vi "SS2 Live_Write HDF5 Header.vi"(8 "error in (no error)":errorcluster, 10 "Current Data Set":i32, 11 "ref in":T1 format="%.0x") -> (0 "Error Out":errorcluster, 1 "Notebook Message":string, 2 "# Image Sets":u32, 3 "ref out":T1 format="%.0x", 5 "# Data Sets":i32)   [LabVIEW 2019]
uses:
  <vilib>/addons/h5labview2/base/hid_t.ctl
  SS2 Live_Settings List.ctl
  SS2 Live_File Information.ctl
  SS2 Live_Image ROI Information.ctl
  Phasor/Image Binning Options.ctl
  SS2 DAQ Parameters 2.ctl
  SS2 Gate Definition.ctl
  Phasor/Fluorescence Lifetime Parameters.ctl
  <vilib>/addons/h5labview2/base/lib_path.vi
  <vilib>/addons/h5labview2/base/H5Equery.vi
  <vilib>/addons/h5labview2/dataset/H5Dwrite.llb/H5Dwrite.xnode
  <vilib>/addons/h5labview2/group/H5G.lvlib
  Variant/Variant to Data/Variant to Data.lvlib
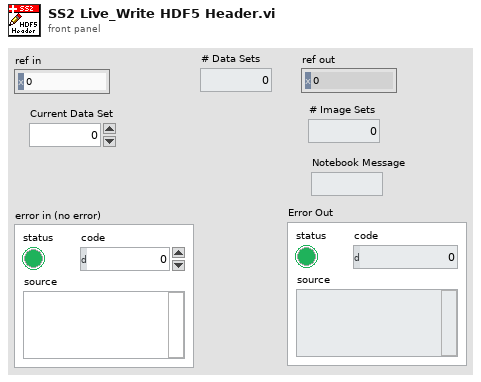
[diagram p1: front panel]
types:
  T1 = typedef "hid_t.ctl" = i32
  T2 = typedef "SS2 Live_Settings List.ctl" = enum16{"FPGA:Bitfile Path", "FPGA:Bitfile Version", "Acquisition Parameters:SS2 DAQ Parameters", "Acquisition Parameters:Gate Configuration Array", "Acquisition Parameters:Buffer Size (# Gates)", "File Information:File Information", "File Information:# Datasets in Series", "Image Parameters:Image ROI Information", "Image Parameters:Image Binning Options", "UI Parameters:Histogram Bins Number"}
  T3 = typedef "SS2 Live_File Information.ctl" = cluster{"File Folder":path, "File Name":string, "File Index":u32, "Author":string, "Sample":string, "Compression":bool}
  T4 = typedef "Image Binning Options.ctl" = cluster{"Use Image Binning":bool, "X Bin":i32, "Y Bin":i32}
  T5 = typedef "SS2 Live_Image ROI Information.ctl" = cluster{"Save ROI Only":bool, "Left":u16, "Top":u16, "Right":u16, "Bottom":u16, "Use Current ROI":bool}
  T6 = typedef "Fluorescence Lifetime Parameters.ctl" = cluster{"# Pixel X":i32, "# Pixel Y":i32, "# Gates":i32, "# Datasets":i32, "Exposure/Gate":dbl[unit], "Macrotime Gate Separation":dbl[unit], "Nanotime Gate Separation":dbl[unit], "Gate Duration":dbl[unit], "Laser Period":dbl[unit]}
  T7 = typedef "SS2 DAQ Parameters 2.ctl" = cluster{"10 bits":bool, "# Exposure Sequences":u32, "# 1-bit Frame per Gate":u32, "Gate Shift":u32, "# Gates per Set":u32, "# Sets":u32, "Laser Period":dbl[unit], "Gate Offset":u32, "Auto-adjust Gate Offset":bool, "Gate Definition":T8}
  T8 = typedef "SS2 Gate Definition.ctl" = cluster{"gs_psincdec_0":u32, "gs_psincdec_1":u32, "gs_psincdec_2":u32, "gs_psincdec_3":u32, "gs_no_shift_adj_1":u32, "gs_no_shift_adj_2":u32, "gs_no_shift_adj_3":u32}
  T9 = typedef "SS2 Live_Gate Characteristics.ctl" = cluster{"Predicted Gate Width":dbl[unit], "Gate Image Duration":dbl[unit], "Gate Image Exposure":dbl[unit], "Gate Shift":dbl[unit], "Gate Images Span":dbl[unit]}
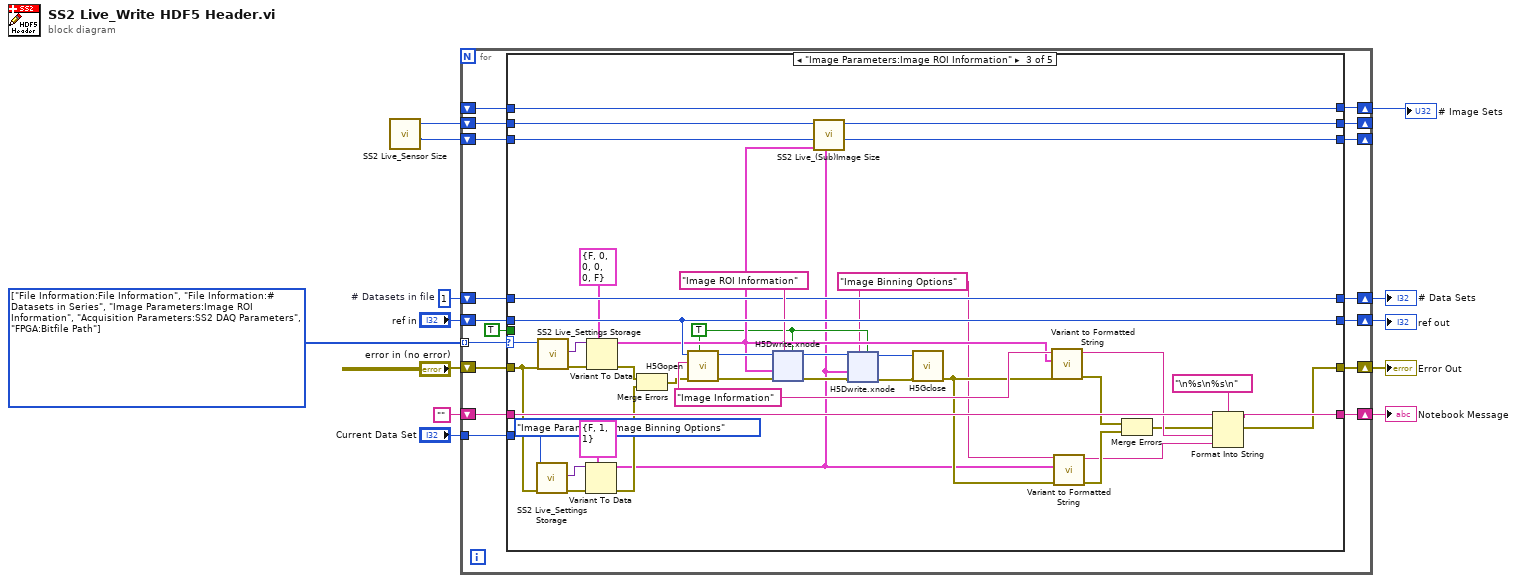
[diagram p0: block diagram]
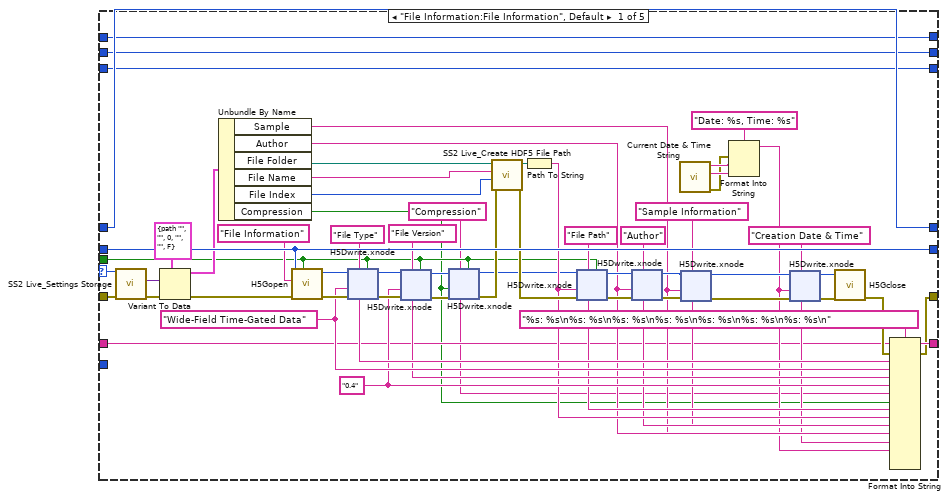
[diagram p2: hidden frame]
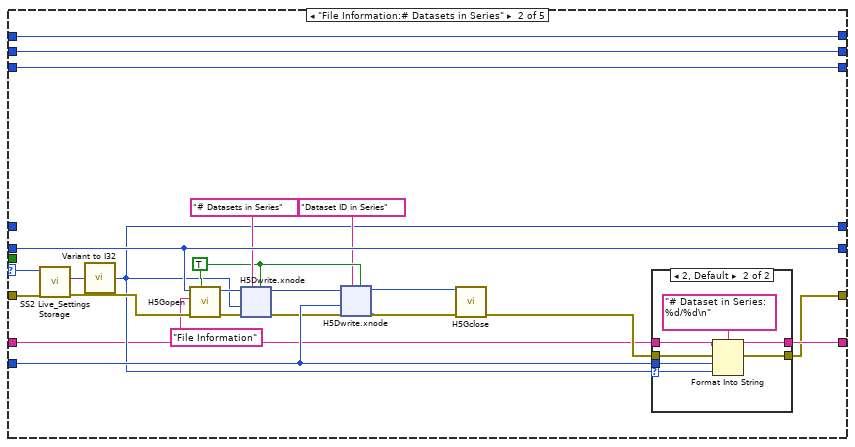
[diagram p3: hidden frame]
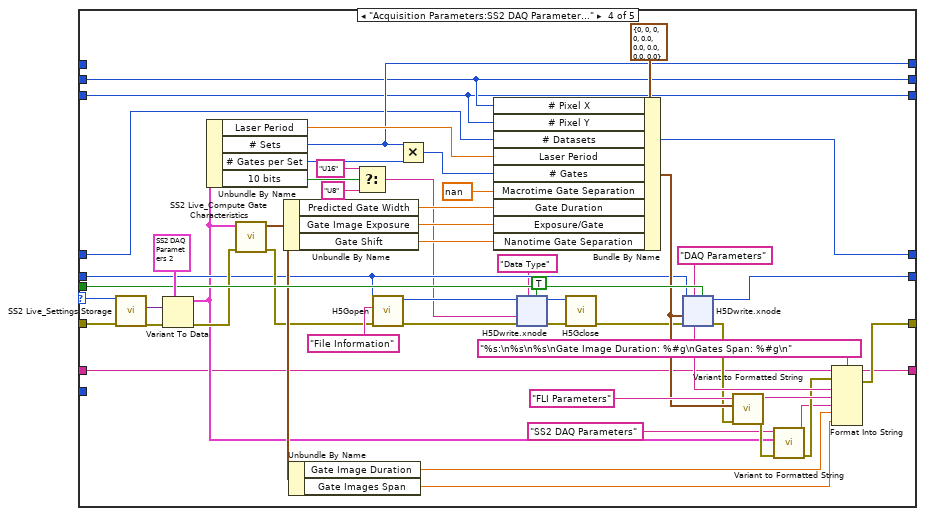
[diagram p5: hidden frame]
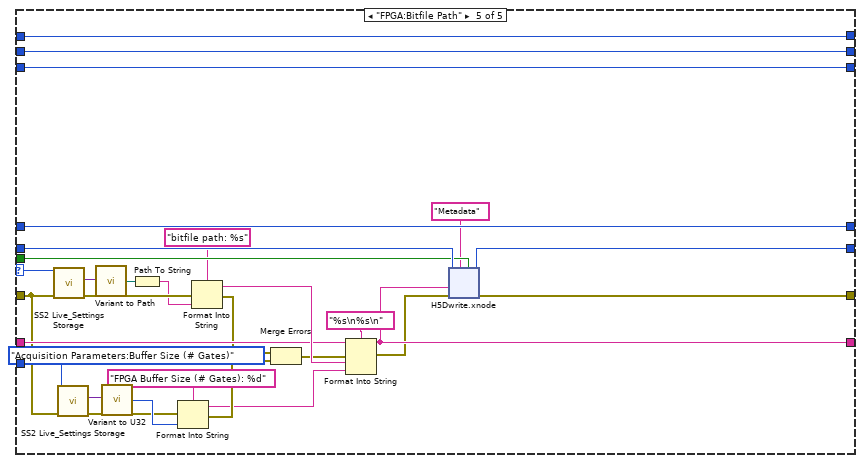
[diagram p6: hidden frame]
diagram:
  w8 = 1  # # Datasets in file
  w13 = T2[] [enum."File Information:File Information", enum."File Information:# Datasets in Series", enum."Image Parameters:Image ROI Information", enum."Acquisition Parameters:SS2 DAQ Parameters", enum."FPGA:Bitfile Path"] items=["FPGA:Bitfile Path", "FPGA:Bitfile Version", "Acquisition Parameters:SS2 DAQ Parameters", "Acquisition Parameters:Gate Configuration Array", "Acquisition Parameters:Buffer Size (# Gates)", "File Information:File Information", "File Information:# Datasets in Series", "Image Parameters:Image ROI Information", "Image Parameters:Image Binning Options", "UI Parameters:Histogram Bins Number"] ("Array")
  n1 = call "SS2 Live_Sensor Size.vi"() -> ("Y size"=w1:i32, "X size"=w2:i32)  [unwired: 10 in]
  n2 = for {
    tunnel: w13 -> [w30] mode=indexing
    shift-right: [w26] -> w10
    shift-left: "ref in" -> [w28]
    shift-right: [w27] -> w9
    shift-left: "error in (no error)" -> [w29]
    shift-right: [w23] -> w5
    shift-left: w8 -> [w22]
    tunnel: "Current Data Set" -> [w21]
    shift-right: [w20] -> w6
    shift-left: _ -> [w19]
    shift-right: [w24] -> w3
    shift-left: "" -> [w18]
    shift-right: [w16] -> _
    shift-left: w2 -> [w17]
    shift-right: [w14] -> _
    shift-left: w1 -> [w15]
    n3 = case shown="\"Image Parameters:Image ROI Information\"" w30 {
      selector: w30 -> [w84 w242 w331 w416 w488]
      tunnel: w29 -> [w85 w243 w302 w417 w466]
      tunnel: w28 -> [w79 w236 w329 w387 w485]
      tunnel: [w43 w239 w317 w404 w470] -> w27
      tunnel: [w79 w236 w329 w415 w484] -> w26
      tunnel: TRUE ("replace? (F)") -> [w33 _ _ w414 w483]
      tunnel: [w46 w240 w319 w374 w473] -> w24
      tunnel: [w42 w223 w324 w372 w477] -> w23
      tunnel: w22 -> [w42 _ w324 w372 w477]
      tunnel: w21 -> [_ w235 _ _ _]
      tunnel: [w41 w224 w325 w380 w476] -> w20
      tunnel: w19 -> [w41 w224 w325 _ w476]
      tunnel: w18 -> [w40 w222 w320 w373 w474]
      tunnel: [w39 w221 w312 w371 w469] -> w16
      tunnel: w17 -> [w39 w221 w313 w371 w469]
      tunnel: [w38 w220 w310 w370 w468] -> w14
      tunnel: w15 -> [w38 w220 w311 w370 w468]
      frame "File Information:File Information", Default {
        w32 = "Compression" ("dataset name")
        w48 = "Creation Date & Time" ("dataset name")
        w50 = "Sample Information" ("dataset name")
        w52 = "Author" ("dataset name")
        w54 = "File Path" ("dataset name")
        w57 = "Wide-Field Time-Gated Data" ("dataset name")
        w58 = "File Type" ("dataset name")
        w55 = "0.4" ("dataset name")
        w56 = "File Version" ("dataset name")
        n4 = call "SS2 Live_Settings Storage.vi"("Error In"=w85, "Settings List"=w84) -> ("Error Out"=w88:errorcluster, "Variant Data out"=w87:variant)  [unwired: 8 in]
        n5 = Variant To Data(error in=w88, type=T3 {"File Folder"=path "", "File Name"="", "File Index"=0, "Author"="", "Sample"="", "Compression"=FALSE} ("File Information"), Variant=w87) -> (data=w77:T3, error out=w78:errorcluster)
        n6 = Unbundle By Name(w77) -> ("Sample"=w49:string, "Author"=w51:string, "File Folder"=w76:path, "File Name"=w75:string, "File Index"=w74:u32, "Compression"=w31:bool)
        n7 = call <vilib>:"H5Gopen.vi"("create? (F)"=w33, "error in (no error)"=w78, "name"="File Information", "ref in"=w79) -> ("error out"=w82:errorcluster, "group out"=w83:T1)  [unwired: 6 in]
        n8 = xnode "H5Dwrite.xnode"("replace? (F)"=w33, "dataset name"=w58, "error in (no error)"=w82, "data"=w57, "ref in"=w83) -> ("error out"=w81:errorcluster, "ref out"=w80:i32)  [unwired: 2 in, 1 out]
        n9 = xnode "H5Dwrite.xnode"("replace? (F)"=w33, "dataset name"=w56, "error in (no error)"=w81, "data"=w55, "ref in"=w80) -> ("error out"=w37:errorcluster, "ref out"=w35:i32)  [unwired: 2 in, 1 out]
        n10 = xnode "H5Dwrite.xnode"("replace? (F)"=w33, "dataset name"=w32, "error in (no error)"=w37, "data"=w31, "ref in"=w35) -> ("error out"=w36:errorcluster, "ref out"=w34:i32)  [unwired: 2 in, 1 out]
        n11 = call "SS2 Live_Create HDF5 File Path.vi"("error in (no error)"=w36, "File Index"=w74, "File Name"=w75, "File Folder"=w76) -> ("error out"=w73:errorcluster, "File path"=w72:path)  [unwired: 6 in]
        n12 = Path To String(path=w72) -> (string=w53:string)
        n13 = xnode "H5Dwrite.xnode"("replace? (F)"=w33, "dataset name"=w54, "error in (no error)"=w73, "data"=w53, "ref in"=w34) -> ("error out"=w70:errorcluster, "ref out"=w71:i32)  [unwired: 2 in, 1 out]
        n14 = xnode "H5Dwrite.xnode"("dataset name"=w52, "error in (no error)"=w70, "data"=w51, "ref in"=w71) -> ("error out"=w69:errorcluster, "ref out"=w68:i32)  [unwired: 3 in, 1 out]
        n15 = call "Current Date & Time String.vi"() -> ("Error Out"=w62:errorcluster, "time string"=w63:string, "date string"=w64:string)  [unwired: 9 in]
        n16 = xnode "H5Dwrite.xnode"("dataset name"=w50, "error in (no error)"=w69, "data"=w49, "ref in"=w68) -> ("error out"=w67:errorcluster, "ref out"=w66:i32)  [unwired: 3 in, 1 out]
        n17 = Format Into String(format string="Date: %s, Time: %s", error in=w62, w64, w63) -> (resulting string=w47:string)  [unwired: 1 in, 1 out]
        n18 = xnode "H5Dwrite.xnode"("dataset name"=w48, "error in (no error)"=w67, "data"=w47, "ref in"=w66) -> ("error out"=w45:errorcluster, "ref out"=w65:i32)  [unwired: 3 in, 1 out]
        n19 = call <vilib>:"H5Gclose.vi"("error in (no error)"=w45, "group in"=w65) -> ("error out"=w44:errorcluster)  [unwired: 9 in]
        n20 = Format Into String(format string="%s: %s\n%s: %s\n%s: %s\n%s: %s\n%s: %s\n%s: %s\n%s: %s\n", initial string=w40, error in=w44, w58, w57, w56, w55, w32, w31, w54, w53, w52, w51, w50, w49, w48, w47) -> (resulting string=w46:string, error out=w43:errorcluster)
      }
      frame "File Information:# Datasets in Series" {
        w226 = TRUE ("replace? (F)")
        n21 = call "SS2 Live_Settings Storage.vi"("Error In"=w243, "Settings List"=w242) -> ("Error Out"=w238:errorcluster, "Variant Data out"=w241:variant)  [unwired: 8 in]
        n22 = call "Variant to I32.vi"("Variant"=w241) -> ("Value"=w223:i32)  [unwired: 8 in]
        n23 = call <vilib>:"H5Gopen.vi"("create? (F)"=w226, "error in (no error)"=w238, "name"="File Information", "ref in"=w236) -> ("error out"=w233:errorcluster, "group out"=w234:T1)  [unwired: 6 in]
        n24 = xnode "H5Dwrite.xnode"("replace? (F)"=w226, "dataset name"="# Datasets in Series" ("name"), "error in (no error)"=w233, "data"=w223, "ref in"=w234) -> ("error out"=w230:errorcluster, "ref out"=w228:i32)  [unwired: 2 in, 1 out]
        n25 = xnode "H5Dwrite.xnode"("replace? (F)"=w226, "dataset name"="Dataset ID in Series" ("name"), "error in (no error)"=w230, "data"=w235, "ref in"=w228) -> ("error out"=w229:errorcluster, "ref out"=w227:i32)  [unwired: 2 in, 1 out]
        n26 = call <vilib>:"H5Gclose.vi"("error in (no error)"=w229, "group in"=w227) -> ("error out"=w237:errorcluster)  [unwired: 9 in]
        n27 = case shown="2, Default" w223 {
          selector: w223 -> [_ w286]
          tunnel: [w282 w289] -> w240
          tunnel: w237 -> [w283 w288]
          tunnel: [w283 w287] -> w239
          tunnel: w235 -> [_ w285]
          tunnel: w222 -> [w282 w284]
          frame 0, 1 {
          }
          frame 2, Default {
            n28 = Format Into String(format string="# Dataset in Series: %d/%d\n", initial string=w284, error in=w288, w285, w286) -> (resulting string=w289:string, error out=w287:errorcluster)
          }
        }
      }
      frame "Image Parameters:Image ROI Information" {
        w294 = "Image Binning Options" ("name")
        w304 = TRUE ("replace? (F)")
        w316 = "Image Information" ("name")
        n29 = call "SS2 Live_Settings Storage.vi"("Error In"=w302, "Settings List"=SS2_Live_Settings_List."Image Parameters:Image Binning Options") -> ("Error Out"=w301:errorcluster, "Variant Data out"=w303:variant)  [unwired: 8 in]
        n30 = call "SS2 Live_Settings Storage.vi"("Error In"=w302, "Settings List"=w331) -> ("Error Out"=w330:errorcluster, "Variant Data out"=w322:variant)  [unwired: 8 in]
        n31 = Variant To Data(error in=w301, type=T4 {"Use Image Binning"=FALSE, "X Bin"=1, "Y Bin"=1} ("Image Binning Options"), Variant=w303) -> (data=w295:T4, error out=w298:errorcluster)
        n32 = Variant To Data(error in=w330, type=T5 {"Save ROI Only"=FALSE, "Left"=0, "Top"=0, "Right"=0, "Bottom"=0, "Use Current ROI"=FALSE} ("Image Information"), Variant=w322) -> (data=w309:T5, error out=w323:errorcluster)
        n33 = Merge Errors(w323, w298) -> (w299:errorcluster)
        n34 = call <vilib>:"H5Gopen.vi"("create? (F)"=w304, "error in (no error)"=w299, "name"=w316, "ref in"=w329) -> ("error out"=w327:errorcluster, "group out"=w328:T1)  [unwired: 6 in]
        n35 = xnode "H5Dwrite.xnode"("replace? (F)"=w304, "dataset name"="Image ROI Information" ("name"), "error in (no error)"=w327, "data"=w309, "ref in"=w328) -> ("error out"=w308:errorcluster, "ref out"=w306:i32)  [unwired: 2 in, 1 out]
        n36 = call "SS2 Live_(Sub)Image Size.vi"("Image Binning Options"=w295, "Image Information"=w309, "# Pixel Y in"=w311, "# Pixel X in"=w313) -> ("# Pixel Y out"=w310:i32, "# Pixel X out"=w312:i32)  [unwired: 6 in]
        n37 = xnode "H5Dwrite.xnode"("replace? (F)"=w304, "dataset name"=w294, "error in (no error)"=w308, "data"=w295, "ref in"=w306) -> ("error out"=w307:errorcluster, "ref out"=w305:i32)  [unwired: 2 in, 1 out]
        n38 = call <vilib>:"H5Gclose.vi"("error in (no error)"=w307, "group in"=w305) -> ("error out"=w296:errorcluster)  [unwired: 9 in]
        n39 = call "Variant to Formatted String.vi"("Error In"=w296, "Variant"=w309, "Label"=w316) -> ("Error Out"=w318:errorcluster, "String"=w315:string)  [unwired: 7 in]
        n40 = call "Variant to Formatted String.vi"("Error In"=w296, "Variant"=w295, "Label"=w294) -> ("Error Out"=w292:errorcluster, "String"=w291:string)  [unwired: 7 in]
        n41 = Merge Errors(w318, w292) -> (w293:errorcluster)
        n42 = Format Into String(format string="\n%s\n%s\n", initial string=w320, error in=w293, w315, w291) -> (resulting string=w319:string, error out=w317:errorcluster)
      }
      frame "Acquisition Parameters:SS2 DAQ Parameters" {
        w409 = "DAQ Parameters" ("dataset name")
        n43 = call "SS2 Live_Settings Storage.vi"("Error In"=w417, "Settings List"=w416) -> ("Error Out"=w420:errorcluster, "Variant Data out"=w419:variant)  [unwired: 8 in]
        n44 = Variant To Data(error in=w420, type=T7 {"10 bits"=FALSE, "# Exposure Sequences"=0, "# 1-bit Frame per Gate"=0, "Gate Shift"=0, "# Gates per Set"=0, "# Sets"=1, "Laser Period"=0.0, "Gate Offset"=0, "Auto-adjust Gate Offset"=FALSE, "Gate Definition"={"gs_psincdec_0"=0, "gs_psincdec_1"=0, "gs_psincdec_2"=0, "gs_psincdec_3"=0, "gs_no_shift_adj_1"=0, "gs_no_shift_adj_2"=0, "gs_no_shift_adj_3"=0}} ("SS2 DAQ Parameters"), Variant=w419) -> (data=w376:T7, error out=w402:errorcluster)
        n45 = Unbundle By Name(w376) -> ("Laser Period"=w399:dbl[unit], "# Sets"=w380:u32, "# Gates per Set"=w412:u32, "10 bits"=w385:bool)
        n46 = call "SS2 Live_Compute Gate Characteristics.vi"("Error In"=w402, "SS2 DAQ Parameters"=w376) -> ("Error Out"=w392:errorcluster, "Gate Characteristics"=w397:T9)  [unwired: 8 in]
        n47 = Unbundle By Name(w397) -> ("Predicted Gate Width"=w401:dbl[unit], "Gate Image Exposure"=w400:dbl[unit], "Gate Shift"=w398:dbl[unit])
        n48 = Unbundle By Name(w397) -> ("Gate Image Duration"=w396:dbl[unit], "Gate Images Span"=w395:dbl[unit])
        n49 = Select(t="U16" ("name"), s=w385, f="U8" ("name")) -> (s? t:f=w381:string)
        n50 = call <vilib>:"H5Gopen.vi"("error in (no error)"=w392, "name"="File Information", "ref in"=w387) -> ("error out"=w391:errorcluster, "group out"=w394:T1)  [unwired: 7 in]
        n51 = Multiply(x=w380, y=w412) -> (x*y=w411:u32)
        n52 = Bundle By Name(cluster=T6 {"# Pixel X"=0, "# Pixel Y"=0, "# Gates"=0, "# Datasets"=0, "Exposure/Gate"=0.0, "Macrotime Gate Separation"=0.0, "Nanotime Gate Separation"=0.0, "Gate Duration"=0.0, "Laser Period"=0.0} ("FLI Parameters"), "# Pixel X"=w371, "# Pixel Y"=w370, "# Datasets"=w372, "Laser Period"=w399, "# Gates"=w411, "Macrotime Gate Separation"=dbl[unit] nan, "Gate Duration"=w401, "Exposure/Gate"=w400, "Nanotime Gate Separation"=w398) -> (w407:T6)
        n53 = xnode "H5Dwrite.xnode"("replace? (F)"=TRUE, "dataset name"="Data Type", "error in (no error)"=w391, "data"=w381, "ref in"=w394) -> ("error out"=w390:errorcluster, "ref out"=w388:i32)  [unwired: 2 in, 1 out]
        n54 = call <vilib>:"H5Gclose.vi"("error in (no error)"=w390, "group in"=w388) -> ("error out"=w389:errorcluster)  [unwired: 9 in]
        n55 = xnode "H5Dwrite.xnode"("replace? (F)"=w414, "dataset name"=w409, "error in (no error)"=w389, "data"=w407, "ref in"=w387) -> ("error out"=w405:errorcluster, "ref out"=w415:i32)  [unwired: 2 in, 1 out]
        n56 = call "Variant to Formatted String.vi"("Error In"=w405, "Variant"=w407, "Label"="FLI Parameters") -> ("Error Out"=w379:errorcluster, "String"=w406:string)  [unwired: 7 in]
        n57 = call "Variant to Formatted String.vi"("Error In"=w379, "Variant"=w376, "Label"="SS2 DAQ Parameters") -> ("Error Out"=w378:errorcluster, "String"=w377:string)  [unwired: 7 in]
        n58 = Format Into String(format string="%s:\n%s\n%s\nGate Image Duration: %#g\nGates Span: %#g\n", initial string=w373, error in=w378, w409, w406, w377, w396, w395) -> (resulting string=w374:string, error out=w404:errorcluster)
      }
      frame "FPGA:Bitfile Path" {
        n59 = call "SS2 Live_Settings Storage.vi"("Error In"=w466, "Settings List"=w488) -> ("Error Out"=w482:errorcluster, "Variant Data out"=w487:variant)  [unwired: 8 in]
        n60 = call "SS2 Live_Settings Storage.vi"("Error In"=w466, "Settings List"=SS2_Live_Settings_List."Acquisition Parameters:Buffer Size (# Gates)") -> ("Error Out"=w463:errorcluster, "Variant Data out"=w465:variant)  [unwired: 8 in]
        n61 = call "Variant to Path.vi"("Variant"=w487) -> ("Path"=w486:path)  [unwired: 8 in]
        n62 = call "Variant to U32.vi"("Variant"=w465) -> ("Value"=w464:u32)  [unwired: 8 in]
        n63 = Path To String(path=w486) -> (string=w481:string)
        n64 = Format Into String(format string="FPGA Buffer Size (# Gates): %d", error in=w463, w464) -> (resulting string=w459:string, error out=w461:errorcluster)  [unwired: 1 in]
        n65 = Format Into String(format string="bitfile path: %s", error in=w482, w481) -> (resulting string=w478:string, error out=w472:errorcluster)  [unwired: 1 in]
        n66 = Merge Errors(w472, w461) -> (w462:errorcluster)
        n67 = Format Into String(format string="%s\n%s\n", initial string=w474, error in=w462, w478, w459) -> (resulting string=w473:string, error out=w471:errorcluster)
        n68 = xnode "H5Dwrite.xnode"("replace? (F)"=w483, "dataset name"="Metadata", "error in (no error)"=w471, "data"=w473, "ref in"=w485) -> ("error out"=w470:errorcluster, "ref out"=w484:T1)  [unwired: 2 in, 1 out]
      }
    }
  }
  "ref out" <- w10
  "Error Out" <- w9
  "Notebook Message" <- w3
  "# Image Sets" <- w6
  "# Data Sets" <- w5
